vi "cm2nm_fiducial_index.vi"(1 "Accept_unverified":bool, 2 "CollectionOfPoints":T1[](array[typedef])) -> (0 "Array":i32[](array[numeric]))   [LabVIEW 2011]
uses:
  cm2nm_coordinate_information_v2.ctl
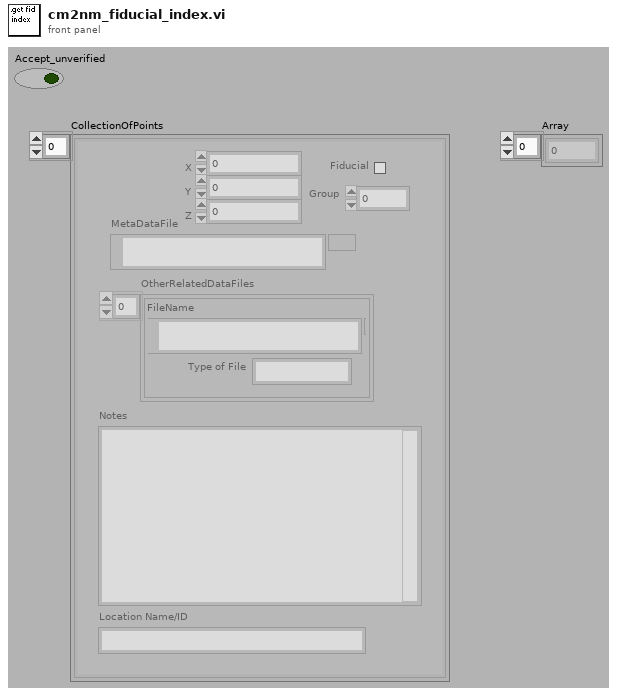
[diagram p1: front panel]
types:
  T1 = typedef "cm2nm_coordinate_information_v2.ctl" = cluster{"MetaDataFile":path, "X":dbl, "Y":dbl, "Z":dbl, "Group":i32, "Rotation":dbl[unit], "Fiducial":bool, "Magnification":dbl, "Working_Distance":dbl, "Notes":string, "Location Name/ID":string, "OtherRelatedDataFiles":cluster{"Type of File":string, "FileName":path}[], "Available":bool}
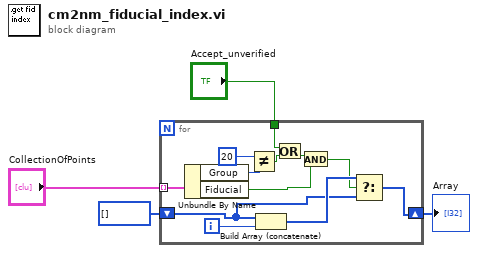
[diagram p0: block diagram]
diagram:
  n1 = for {
    tunnel: "CollectionOfPoints" -> [w16] mode=indexing
    shift-right: [w12] -> w4
    shift-left: i32[] [] -> [w13]
    tunnel: "Accept_unverified" -> [w6]
    i -> [w15]
    n2 = Unbundle By Name(w16) -> ("Group"=w11:i32, "Fiducial"=w9:bool)
    n3 = Not Equal?(x=20, y=w11) -> (x != y?=w5:bool)
    n4 = Build Array (concatenate)(w13, w15) -> (w14:i32[])
    n5 = Or(x=w6, y=w5) -> (x .or. y?=w7:bool)
    n6 = And(x=w7, y=w9) -> (x .and. y?=w8:bool)
    n7 = Select(t=w14, s=w8, f=w13) -> (s? t:f=w12:i32[])
  }
  "Array" <- w4
